vi "SOC_FM Copy Graph to Clipboard.vi"(8 "error in (no error)":errorcluster, 11 "Data":T1={"UI References"={"Exit Ref"=refnum, "Save Ref"=refnum, "Open Ref"=refnum, "Export Ref"=refnum, "Acquire Ref"=refnum, "Configure Ref"=refnum, "Graph Ref"=refnum, "Clear Ref"=refnum, "Analyze Ref"=refnum, "Status Ref"=refnum, "Snapshot Ref"=refnum}, "Graph Data"={"Data"=[], "Annotation List"=[], "Cursor List"=[], "Analysis Data"=[]}, "User Specified"={"Hardware Configuration"={"HW Refnum <Replace Me>"="", "Signal Type <Replace Me>"=enum."Sine Wave"}, "Analysis Configuration"={"Statistics"=TRUE}, "New Data Behavior"=enum."Replace", "Calc PPL Path"=path "", "Calc Plugin Class Qualified Name"="", "Calc Configuration String"=""}, "AbstractCalc"=refnum}) -> (0 "error out":errorcluster)   [LabVIEW 2015]
doc: "Copies an image of the graph to the clipboard."
uses:
  controls/SOC_FM Data.ctl
  PPL/AbstractCalcLib.lvlibp/AbstractCalc/AbstractCalc.lvclass
  controls/SOC_FM UI References.ctl
  controls/SOC_FM Graph Data.ctl
  <vilib>/Utility/miscctls.llb/LVAnnotationListTypeDef.ctl
  <vilib>/Utility/miscctls.llb/LVCursorListTypeDef.ctl
  controls/SOC_FM HW Configuration.ctl
  controls/SOC_FM Simulated Signal Type.ctl
  controls/SOC_FM Analysis Configuration.ctl
  controls/SOC_FM New Data Behavior.ctl
panel:
  # "(Scroll up to see large data cluster)"
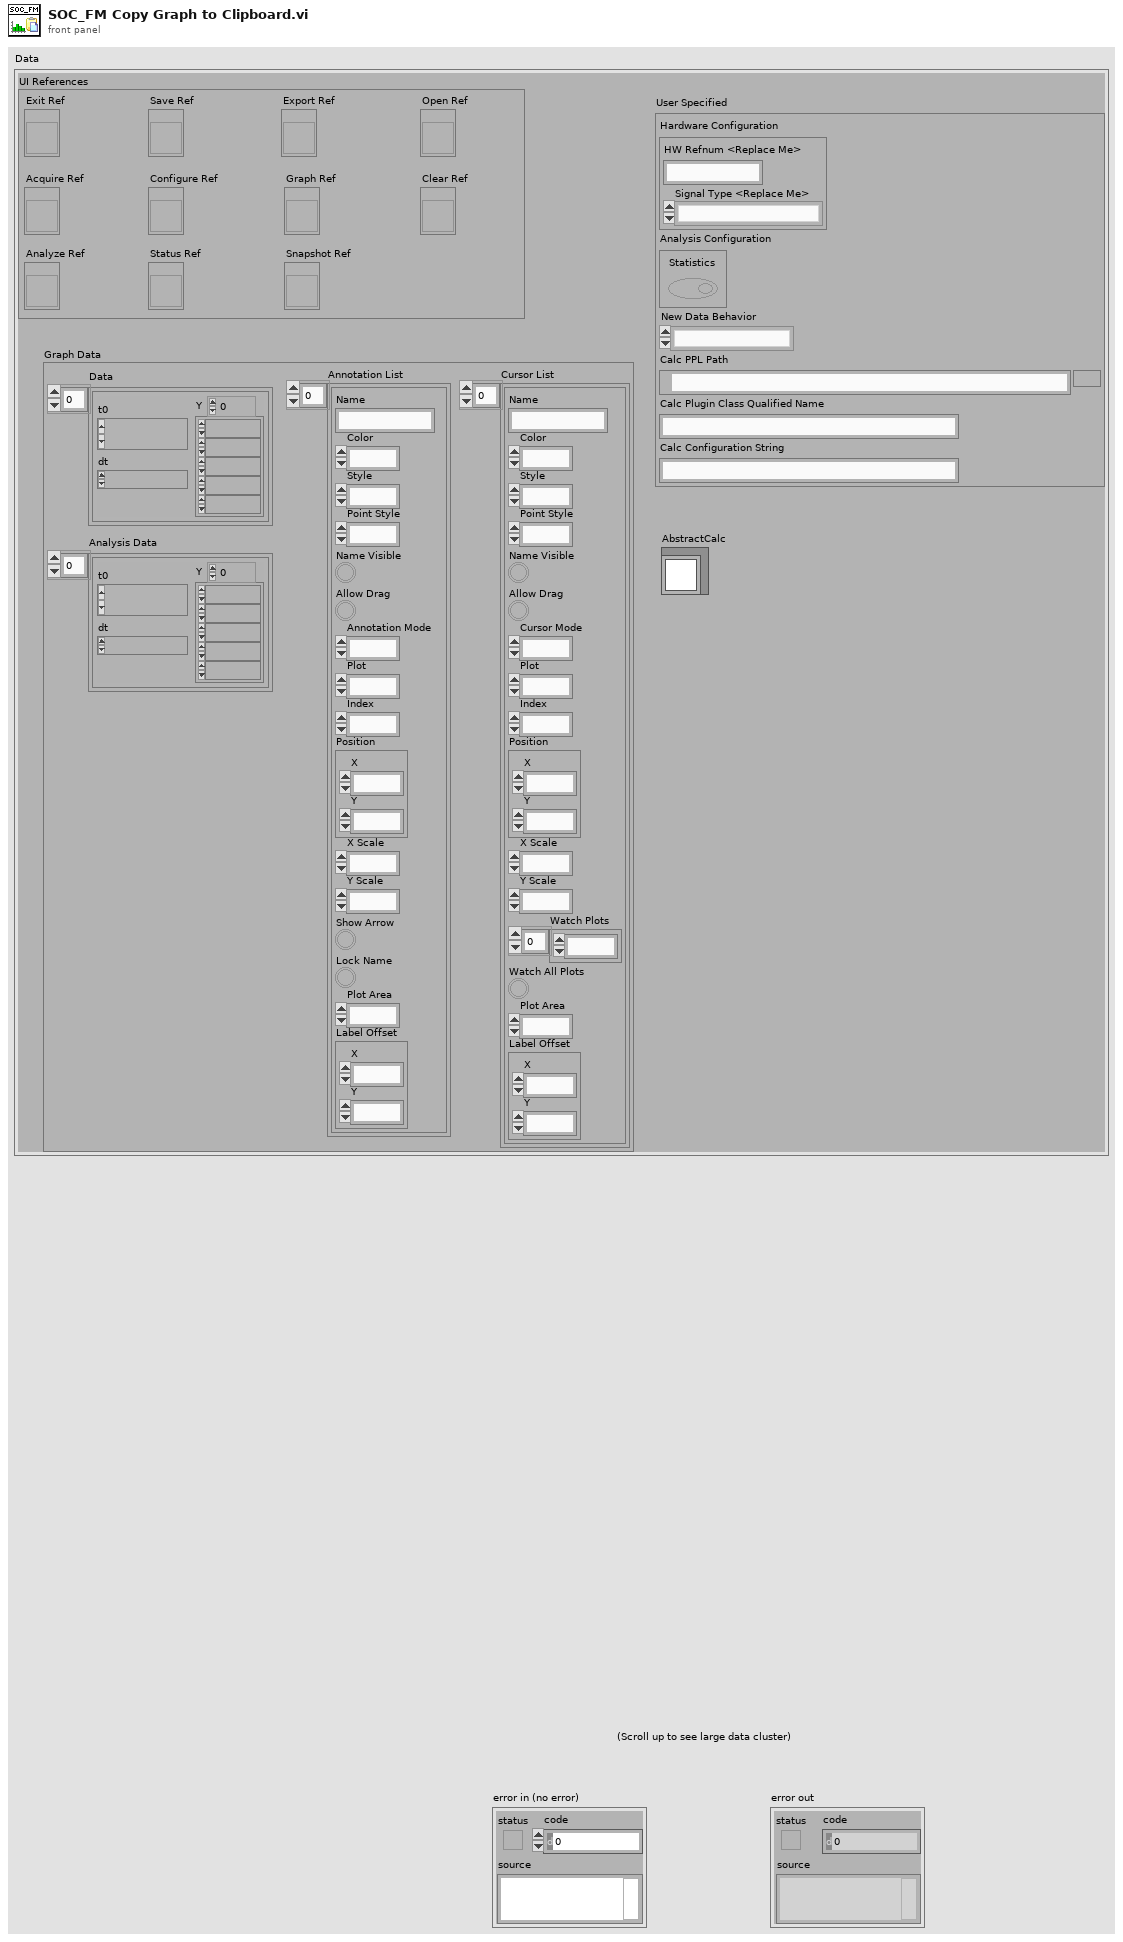
[diagram p1: front panel]
types:
  T1 = typedef "SOC_FM Data.ctl" = cluster{"UI References":T2, "Graph Data":T3, "User Specified":cluster{"Hardware Configuration":T6, "Analysis Configuration":T8, "New Data Behavior":T9, "Calc PPL Path":path, "Calc Plugin Class Qualified Name":string, "Calc Configuration String":string}, "AbstractCalc":refnum<class "AbstractCalc.lvclass">}
  T2 = typedef "SOC_FM UI References.ctl" = cluster{"Exit Ref":refnum<vi>, "Save Ref":refnum<vi>, "Open Ref":refnum<vi>, "Export Ref":refnum<vi>, "Acquire Ref":refnum<vi>, "Configure Ref":refnum<vi>, "Graph Ref":refnum<vi>, "Clear Ref":refnum<vi>, "Analyze Ref":refnum<vi>, "Status Ref":refnum<vi>, "Snapshot Ref":refnum<vi>}
  T3 = typedef "SOC_FM Graph Data.ctl" = cluster{"Data":waveform(dbl)[], "Annotation List":T4, "Cursor List":T5, "Analysis Data":waveform(dbl)[]}
  T4 = typedef "LVAnnotationListTypeDef.ctl" = cluster{"Name":string, "Color":u32, "Style":u8, "Point Style":u8, "Name Visible":bool, "Allow Drag":bool, "Annotation Mode":u32, "Plot":i32, "Index":i32, "Position":cluster{"X":dbl, "Y":dbl}, "X Scale":u32, "Y Scale":u32, "Show Arrow":bool, "Lock Name":bool, "Plot Area":i32, "Label Offset":cluster{"X":dbl, "Y":dbl}}[]
  T5 = typedef "LVCursorListTypeDef.ctl" = cluster{"Name":string, "Color":u32, "Style":u8, "Point Style":u8, "Name Visible":bool, "Allow Drag":bool, "Cursor Mode":u32, "Plot":i32, "Index":i32, "Position":cluster{"X":dbl, "Y":dbl}, "X Scale":u32, "Y Scale":u32, "Watch Plots":i32[], "Watch All Plots":bool, "Plot Area":i32, "Label Offset":cluster{"X":dbl, "Y":dbl}}[]
  T6 = typedef "SOC_FM HW Configuration.ctl" = cluster{"HW Refnum <Replace Me>":string, "Signal Type <Replace Me>":T7}
  T7 = typedef "SOC_FM Simulated Signal Type.ctl" = enum16{"Sine Wave", "Square Wave"}
  T8 = typedef "SOC_FM Analysis Configuration.ctl" = cluster{"Statistics":bool}
  T9 = typedef "SOC_FM New Data Behavior.ctl" = enum16{"Replace", "Overlay", "Append"}
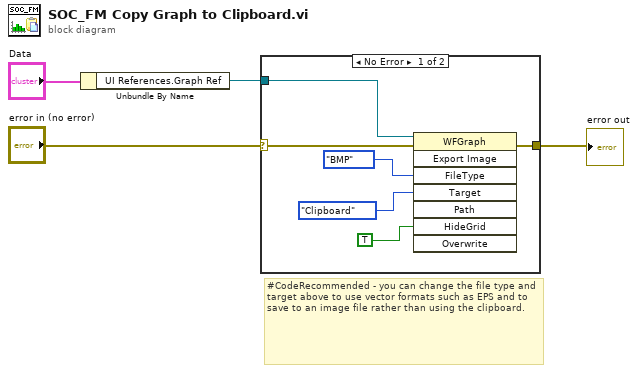
[diagram p0: block diagram]
diagram:
  # "#CodeRecommended - you can change the file type and target above to use vector formats such as EPS and to save to an image file rather than using the clipboard."
  n1 = Unbundle By Name("Data") -> ("UI References.Graph Ref"=w4:refnum<vi>)
  n2 = case shown="No Error" "error in (no error)" {
    selector: "error in (no error)" -> [w5 w11]
    tunnel: w4 -> [w10 _]
    tunnel: [w6 w11] -> w3
    frame No Error {
      n3 = invoke class="WFGraph" method="Export Image"(reference=w10, error in=w5, "FileType"=enum32{"BMP", "EPS", "EMF", "PICT"}."BMP" ("File Type"), "Target"=enum32{"File", "Clipboard"}."Clipboard", "HideGrid"=TRUE ("Hide Grid")) -> (error out=w6:errorcluster)  [unwired: 3 in, 7 out]
    }
    frame Error {
    }
  }
  "error out" <- w3
